vi "Read_Settings.vi"() -> ()   [LabVIEW 2015]
uses:
  <instrlib>/BK Precision 178XB Series/BK Precision 178XB Series.lvlib
panel:
  out "error out":errorcluster
  out "Configured Voltage":dbl format="%#.2g"
  out "VISA resource name out":refnum<visa-resource-name>
  in  "error in (no error)":errorcluster
  in  "VISA resource name":refnum<visa-resource-name>
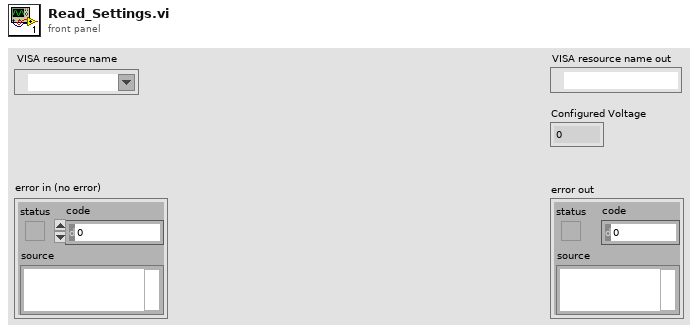
[diagram p1: front panel]
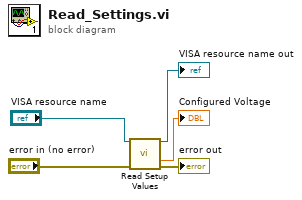
[diagram p0: block diagram]
diagram:
  n1 = call <instrlib>:"Read Setup Values.vi"("VISA resource name"="VISA resource name", "error in (no error)"="error in (no error)") -> ("VISA resource name out"=→"VISA resource name out":refnum<visa-resource-name>, "Configured Voltage"=→"Configured Voltage":dbl, "error out"=→"error out":errorcluster)  [unwired: 9 in, 2 out]
